vi "Interpolate Waveform v3.vi"() -> ()   [LabVIEW 2016]
panel:
  in  "Current dt":dbl
  out "transposed array":dbl[][](array[numeric])
  in  "2D array":dbl[][](array[numeric])
  in  "Match All Data":bool
  out "Resamaple Elements":dbl
  in  "New dt":dbl
  out "resampled waveforms out":waveform(dbl)[](array[waveform])
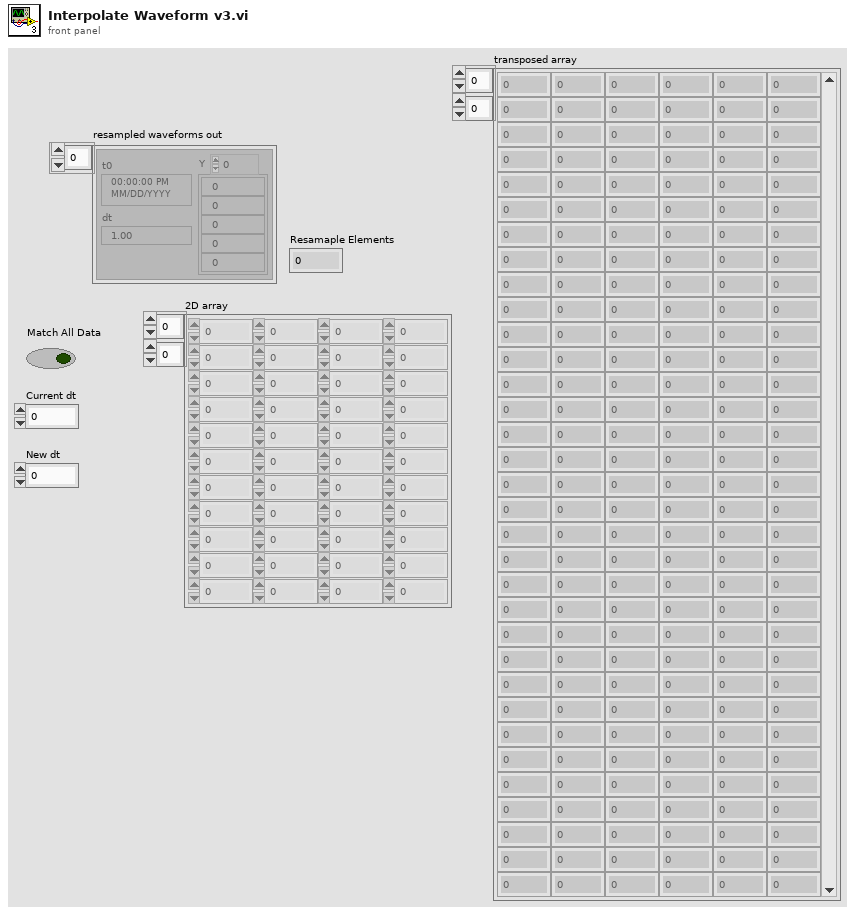
[diagram p1: front panel]
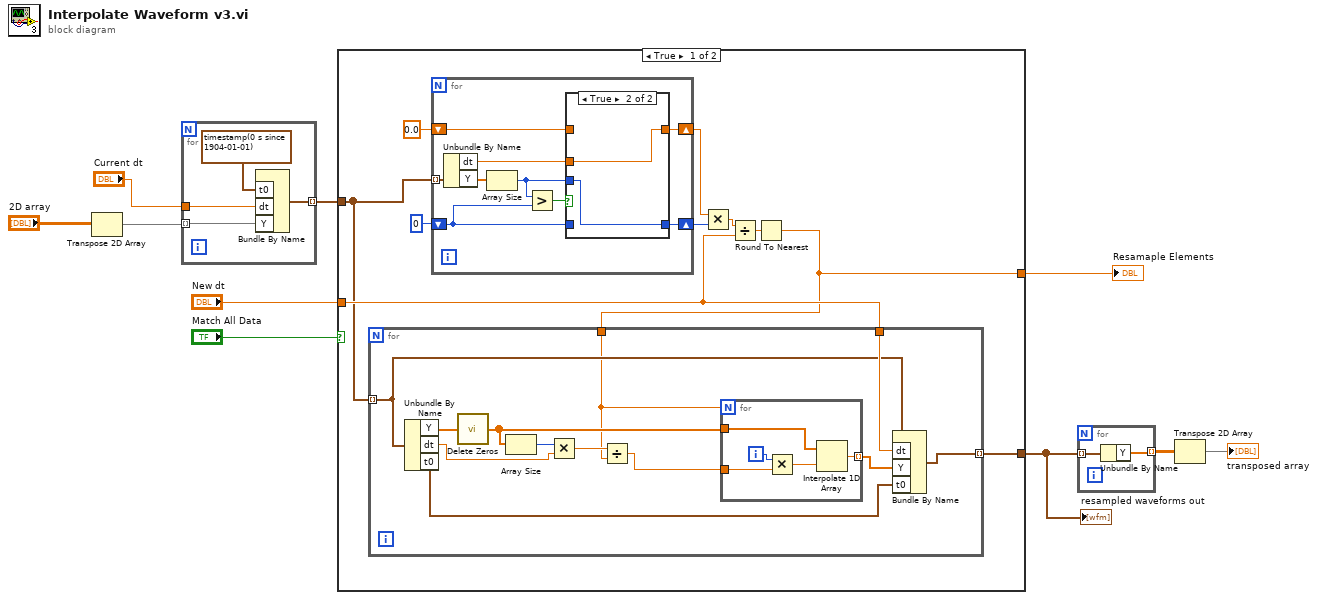
[diagram p0: block diagram]
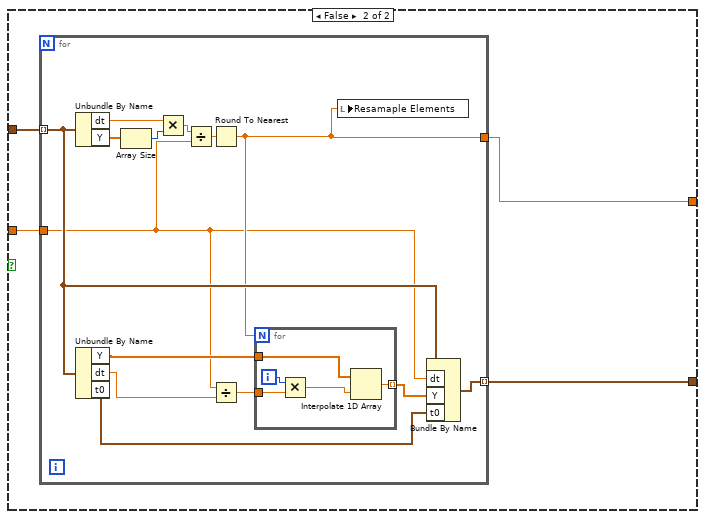
[diagram p3: hidden frame]
diagram:
  n1 = Transpose 2D Array(2D array="2D array") -> (transposed array=w3:dbl[][])
  n2 = for {
    tunnel: w3 -> [w14] mode=indexing
    tunnel: [w13] -> w6 mode=indexing
    tunnel: "Current dt" -> [w11]
    n3 = Bundle By Name("t0"=timestamp(0 s since 1904-01-01), "dt"=w11, "Y"=w14) -> (w13:waveform(dbl))  [unwired: 1 in]
  }
  n4 = case shown="True" "Match All Data" {
    tunnel: "New dt" -> [w23 w56]
    tunnel: [w15 w55] -> w9
    tunnel: w6 -> [w17 w57]
    tunnel: [w16 w58] -> w8
    frame True {
      n5 = for {
        tunnel: w17 -> [w33] mode=indexing
        shift-right: [w28] -> w20
        shift-left: 0 ("size(s)") -> [w30]
        shift-right: [w25] -> w19
        shift-left: 0.0 -> [w27]
        n6 = Unbundle By Name(w33) -> ("dt"=w26:dbl, "Y"=w32:dbl[])
        n7 = Array Size(array=w32) -> (size(s)=w29:i32)
        n8 = Greater?(x=w29, y=w30) -> (0:w31:bool)
        n9 = case shown="True" w31 {
          tunnel: w30 -> [w35 _]
          tunnel: w29 -> [_ w37]
          tunnel: [w35 w37] -> w28
          tunnel: w27 -> [w34 _]
          tunnel: w26 -> [_ w36]
          tunnel: [w34 w36] -> w25
          frame False {
          }
          frame True {
          }
        }
      }
      n10 = Multiply(x=w19, y=w20) -> (x*y=w21:dbl)
      n11 = Divide(x=w21, y=w23) -> (x/y=w18:dbl)
      n12 = Round To Nearest(number=w18) -> (nearest integer value=w15:dbl)
      n13 = for {
        tunnel: w15 -> [w39]
        tunnel: w23 -> [w49]
        tunnel: w17 -> [w47] mode=indexing
        tunnel: [w46] -> w16 mode=indexing
        n14 = Unbundle By Name(w47) -> ("Y"=w44:dbl[], "dt"=w41:dbl, "t0"=w45:timestamp)
        n15 = call "Delete Zeros.vi"("Array In"=w44) -> ("Array Out"=w43:dbl[])
        n16 = Array Size(array=w43) -> (size(s)=w42:i32)
        n17 = Multiply(x=w42, y=w41) -> (x*y=w40:dbl)
        n18 = Divide(x=w40, y=w39) -> (x/y=w38:dbl)
        n19 = for {
          N: w39 -> [_]
          tunnel: w43 -> [w53]
          tunnel: [w52] -> w48 mode=indexing
          tunnel: w38 -> [w50]
          i -> [w54]
          n20 = Multiply(x=w54, y=w50) -> (x*y=w51:dbl)
          n21 = Interpolate 1D Array(1:w51, 2:w53) -> (0:w52:dbl)
        }
        n22 = Bundle By Name(cluster=w47, "dt"=w49, "Y"=w48, "t0"=w45) -> (w46:waveform(dbl))
      }
    }
    frame False {
      n23 = for {
        tunnel: [w70] -> w58 mode=indexing
        tunnel: w57 -> [w66] mode=indexing
        tunnel: w56 -> [w59]
        tunnel: [w60] -> w55
        n24 = Unbundle By Name(w66) -> ("dt"=w62:dbl, "Y"=w65:dbl[])
        n25 = Unbundle By Name(w66) -> ("Y"=w72:dbl[], "dt"=w67:dbl, "t0"=w68:timestamp)
        n26 = Array Size(array=w65) -> (size(s)=w61:i32)
        n27 = Multiply(x=w62, y=w61) -> (x*y=w64:dbl)
        n28 = Divide(x=w64, y=w59) -> (x/y=w63:dbl)
        n29 = Round To Nearest(number=w63) -> (nearest integer value=w60:dbl)
        n30 = Divide(x=w59, y=w67) -> (x/y=w69:dbl)
        n31 = for {
          N: w60 -> [_]
          tunnel: w69 -> [w76]
          tunnel: w72 -> [w75]
          tunnel: [w74] -> w71 mode=indexing
          i -> [w77]
          n32 = Multiply(x=w77, y=w76) -> (x*y=w73:dbl)
          n33 = Interpolate 1D Array(1:w73, 2:w75) -> (0:w74:dbl)
        }
        n34 = local write "Resamaple Elements"(w60) -> ()
        n35 = Bundle By Name(cluster=w66, "dt"=w59, "Y"=w71, "t0"=w68) -> (w70:waveform(dbl))
      }
    }
  }
  "resampled waveforms out" <- w8
  "Resamaple Elements" <- w9
  n36 = for {
    tunnel: w8 -> [w79] mode=indexing
    tunnel: [w78] -> w2 mode=indexing
    n37 = Unbundle By Name(w79) -> ("Y"=w78:dbl[])
  }
  n38 = Transpose 2D Array(2D array=w2) -> (transposed array=→"transposed array":dbl[][])
